vi "仁莫密封检测系统.vi"() -> ()   [LabVIEW 2020]
uses:
  <vilib>/NI/Modbus Library/API/Master/Modbus Master.lvclass
  <vilib>/Utility/file.llb/Read Delimited Spreadsheet (string).vi
  <vilib>/NI/Modbus Library/Transmission Data Unit/RTU/RTU Data Unit.lvclass
  <vilib>/NI/Modbus Library/Master Function Definition/Master Function Definition.lvclass
  <vilib>/NI/Modbus Library/Network Protocol/Network Master/Serial/Serial Master.lvclass
  <vilib>/event_ctls.llb/eventvkey.ctl
panel:
  in  "产品序号":string
  out "MES状态":bool
  out "通讯状态":bool
  out "刷新按钮":bool
  out "参数组别":string
  out "测试时间":string
  out "实时压力":string
  out "泄露压力":string
  out "门限压力":string
  out "目标压力":string
  out "测试 NG":string
  out "测试 OK":string
  out "测试结果":string
  out "测试总量":string
  out "实时压力(图)":dbl(graph)
  in  "清除计数":bool
  in  "设备启动":bool
  out "消息框":string
  in  "设备停止":bool
  in  "阻断通讯":bool=TRUE
  out "运行状态":string
  out "失败原因":string
  in  "Exit":bool
  # "仁 莫 密 封 检 测 系 统"
  # "S"
  # "Pa"
  # "Pa"
  # "Pa"
  # "Pa"
  # "pcs"
  # "pcs"
  # "pcs"
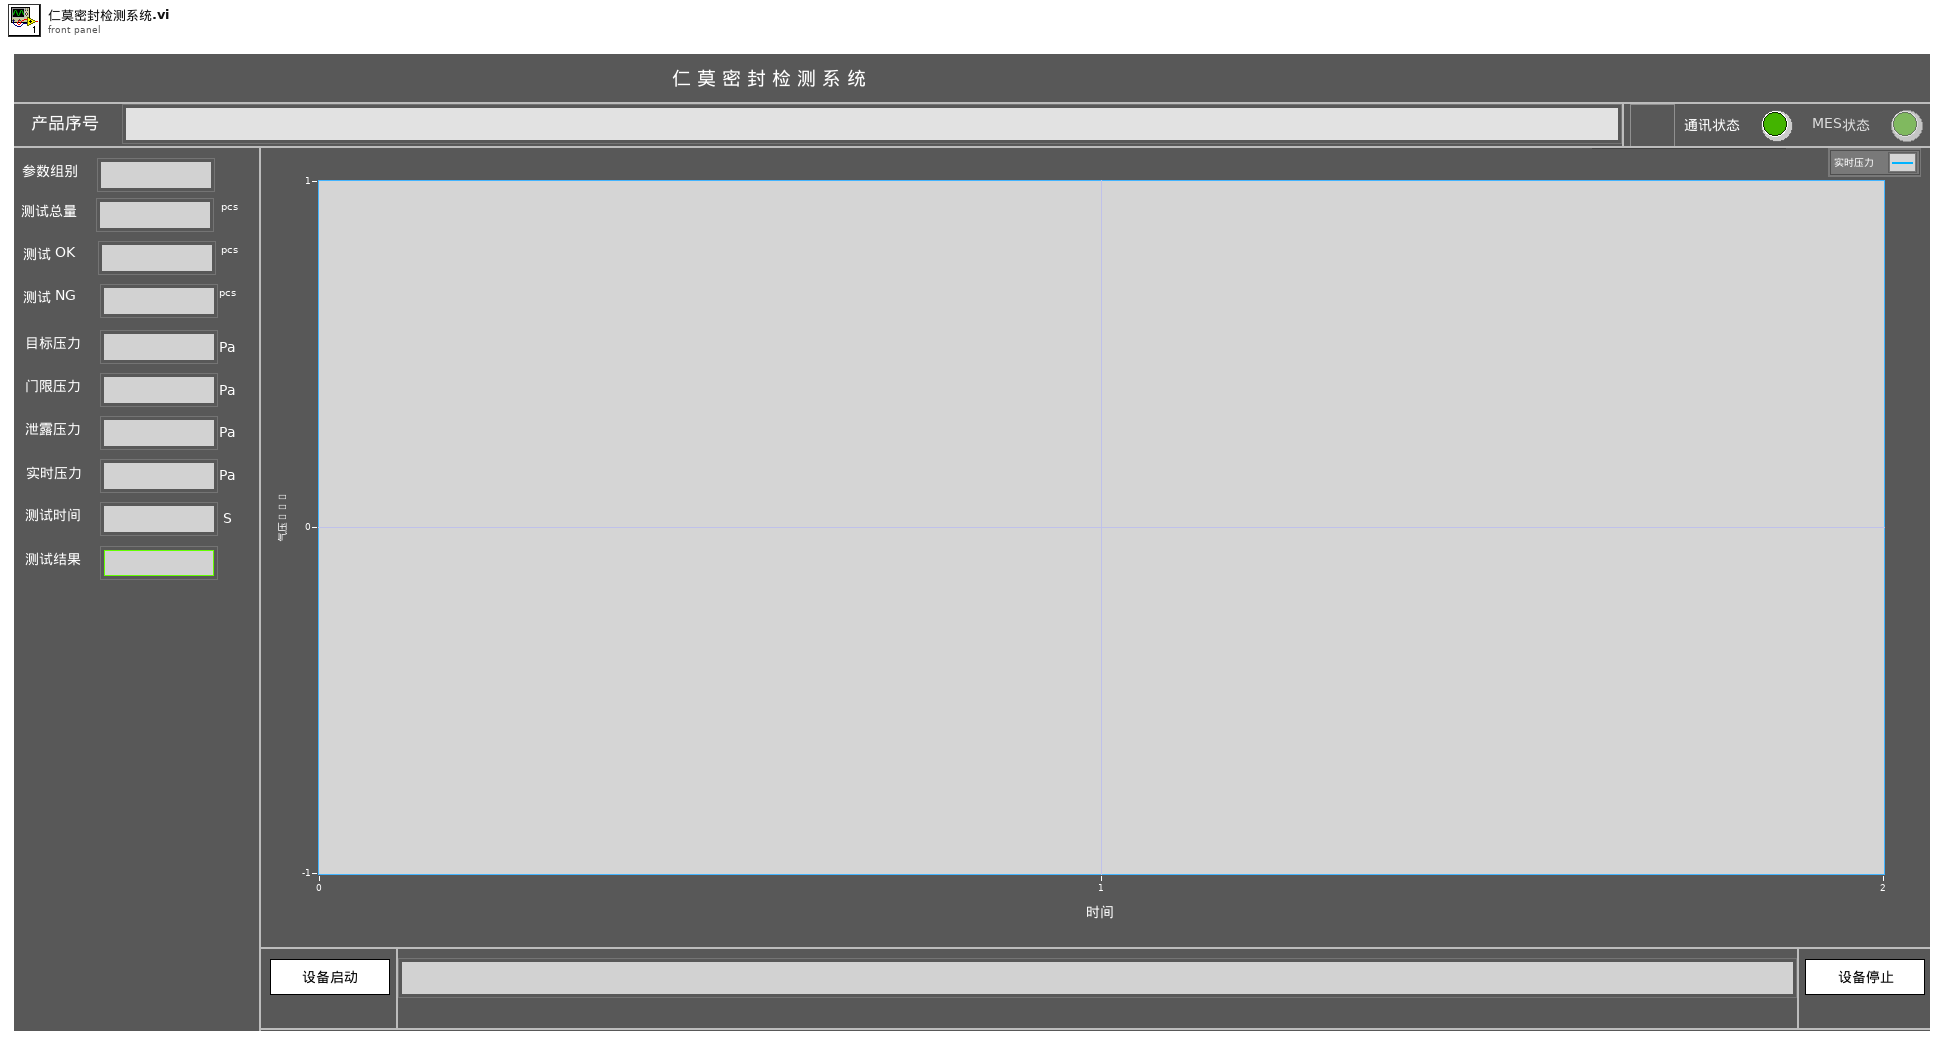
[diagram p1: front panel]
types:
  T1 = typedef "eventvkey.ctl" = enum16{"ASCII", "Enter", "Return", "Shift", "Ctrl", "Alt", "Cmd", "Opt", "Caps", "NumLock", "Clear", "Break", "Up", "Down", "Left", "Right", "Insert", "Delete", "Home", "End", "PageUp", "PageDown", "Escape", "Help", "Pause", "ScrollLock", "F1", "F2", "F3", "F4", "F5", "F6", "F7", "F8", "F9", "F10", "F11", "F12", "F13", "F14", "F15", "F16", "F17", "F18", "F19", "F20", "F21", "F22", "F23", "F24", "Play", "VolumeUp", "VolumeDown", "Mute", "Two Byte Char"}
  T2 = cluster{"地址":u16, "数量":u16, "寄存器值":u16[], "产品总数":string}[]
  T3 = enum32{"Invalid", "Standard", "Closed", "Hidden", "Minimized", "Maximized"}
  T4 = enum32{"invalid app kind", "Development System", "Run Time System", "Student Edition", "Embedded LabVIEW", "Evaluation", "Custom"}
  T5 = cluster{"地址":u16, "数量":u16, "寄存器值":u16[], "名称":string}[]
  T6 = cluster{"读取信息簇":cluster{"地址":u16, "数量":u16, "寄存器值":u16[], "名称":string}, "值解析":string}[]
  T7 = cluster{"温度instance":refnum<class "Modbus Master.lvclass">, "Core":cluster{"Current VI Reference":refnum<vi>, "Close Panel on Exit?":bool}, "serial master instance":refnum<class "Modbus Master.lvclass">, "进站OK":bool, "连接成功":bool, "正在运行":bool, "用户登录":bool, "A读保持寄存器信息组":cluster{"地址":u16, "数量":u16, "寄存器值":u16[], "名称":string}[], "A写入线圈信息组":cluster{"地址":u16, "布尔":bool, "名称":string}[], "A读多组线圈信息组":cluster{"地址":u16, "数量":u16, "名称":string, "线圈组":bool[]}[]}
  T8 = cluster{"连接成功":bool, "MB_实体":refnum<class "Modbus Master.lvclass">}
  T9 = cluster{"地址":u16, "数量":u16, "名称":string, "线圈组":bool[]}[]
  T10 = cluster{"Current VI Reference":refnum<vi>, "Close Panel on Exit?":bool}
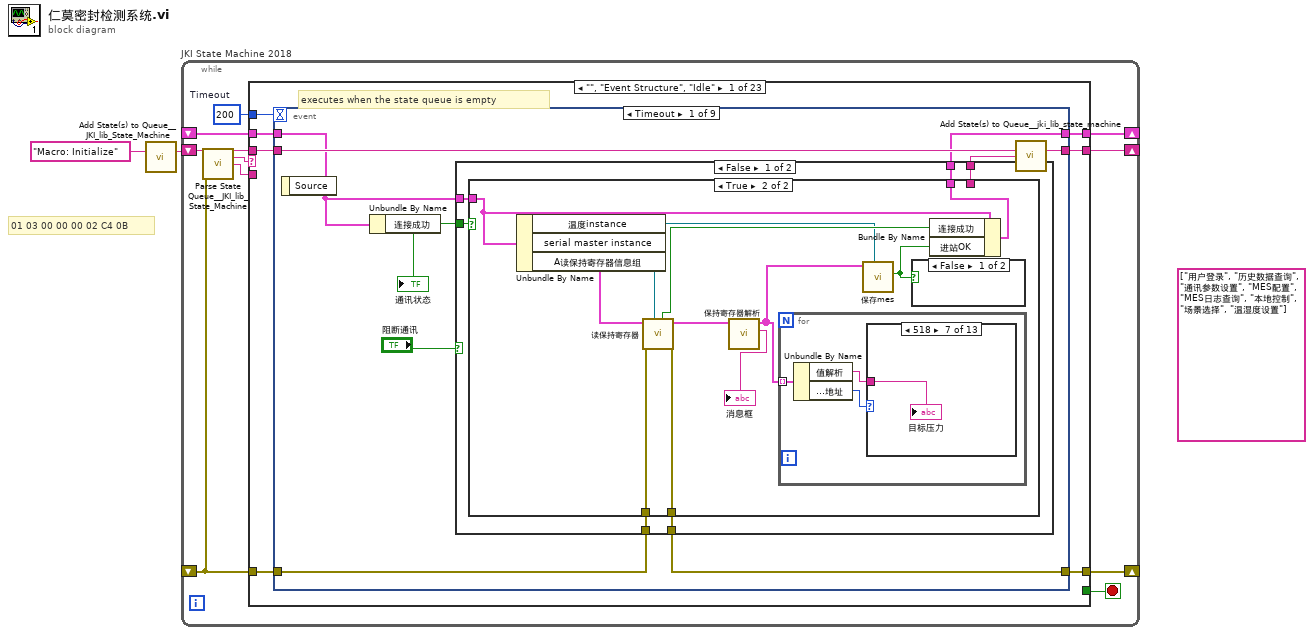
[diagram p0: block diagram]
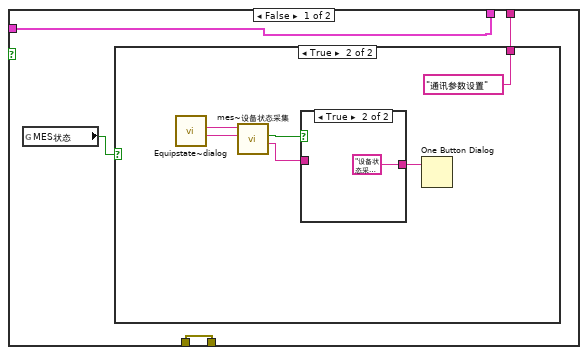
[diagram p2: hidden frame]
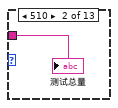
[diagram p7: hidden frame]
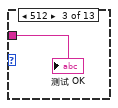
[diagram p8: hidden frame]
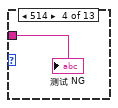
[diagram p9: hidden frame]
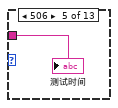
[diagram p10: hidden frame]
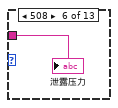
[diagram p11: hidden frame]
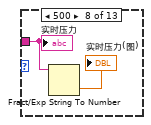
[diagram p12: hidden frame]
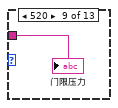
[diagram p13: hidden frame]
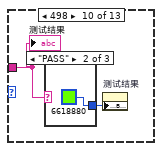
[diagram p14: hidden frame]
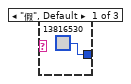
[diagram p15: hidden frame]
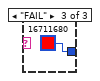
[diagram p16: hidden frame]
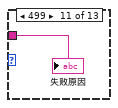
[diagram p17: hidden frame]
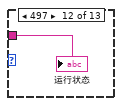
[diagram p18: hidden frame]
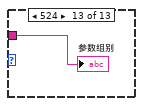
[diagram p19: hidden frame]
diagram:
  (unwired) string[] ["用户登录", "历史数据查询", "通讯参数设置", "MES配置", "MES日志查询", "本地控制", "场景选择", "温湿度设置"] ("L10n_item tags 1")
  # "01 03 00 00 00 02 C4 0B"
  n1 = call <vilib>:"Add State(s) to Queue__JKI_lib_State_Machine.vi"("State(s) in (\"\")"="Macro: Initialize") -> ("States Out"=w2:string)  [unwired: 14 in]
  n2 = while "JKI State Machine 2018" {
    shift-right: [w6] -> _
    shift-left: _ -> [w5]
    shift-right: [w9] -> _
    shift-left: _ -> [w3]
    shift-right: [w8] -> _
    shift-left: w2 -> [w10]
    stop <- w7 stop-if-true
    w4 = 200  # Timeout
    n3 = call <vilib>:"Parse State Queue__JKI_lib_State_Machine.vi"("State Queue"=w10, "Error In (no error)"=w3) -> ("Remaining States"=w12:string, "Current State"=w13:string, "Arguments"=w11:string)  [unwired: 11 in]
    n4 = case shown="\"\", \"Event Structure\", \"Idle\"" w13 {
      selector: w13 -> [_ _ w224 _ _ _ _ _ _ _ _ _ _ _ _ _ _ _ _ _ _ _ _]
      tunnel: w12 -> [w20 w223 w228 w247 w254 w259 w263 w284 w292 w296 w310 w316 w327 w396 w401 w411 w416 w432 w457 w506 w549 w561 w566]
      tunnel: w11 -> [_ _ _ _ _ _ _ _ _ _ _ w311 w321 _ _ _ _ _ _ _ _ _ _]
      tunnel: w5 -> [w18 w220 w226 w240 w251 w257 w260 _ w288 w293 w308 w314 w323 w393 w398 w408 w413 w426 w451 w500 w542 w558 w563]
      tunnel: [w17 w221 w230 w244 errorcluster {"status"=FALSE, "code"=0, "source"=""} ("error out") w256 w261 w281 w289 w294 w307 w312 w324 w394 w399 w409 w414 w422 w454 w503 w546 w559 w564] -> w9
      tunnel: w3 -> [w16 w221 w229 w244 w249 w256 w261 w281 w286 w294 w307 w313 w325 w394 w399 w409 w414 w429 w455 w504 w547 w559 w564]
      tunnel: [w19 w222 w227 w246 w253 w258 w262 w283 w291 w295 w309 w315 w326 w395 w400 w410 w415 w431 w456 w505 w548 w560 w565] -> w8
      tunnel: [_ _ _ _ _ TRUE _ _ _ _ _ _ _ _ _ _ _ _ _ _ _ _ _] -> w7
      tunnel: [w15 w220 w226 w245 w251 w257 w260 w282 w288 w293 w308 w314 w323 w393 w398 w408 w413 w424 w449 w498 w543 w558 w562] -> w6
      tunnel: w4 -> [w14 _ _ _ _ _ _ _ _ _ _ _ _ _ _ _ _ _ _ _ _ _ _]
      frame "", "Event Structure", "Idle" {
        # "executes when the state queue is empty"
        n5 = event shown="[0] Timeout" {
          selector: _ -> [_ _ _ _ _ _ _ _ _]
          dyn-events: _ -> [_ _ _ _ _ _ _ _ _]
          timeout: w14 -> [_ _ _ _ _ _ _ _ _]
          tunnel: w20 -> [w29 w86 w91 w97 w171 w193 w203 w213 w219]
          tunnel: [w28 w85 w90 w96 w170 w193 w202 w212 w218] -> w19
          tunnel: w18 -> [w27 w83 w88 w93 w168 w194 w198 w210 w216]
          tunnel: [w25 w84 w89 w95 w169 w191 w195 w211 w217] -> w17
          tunnel: w16 -> [w26 w84 w89 w95 w169 w191 w196 w211 w217]
          tunnel: [w24 w83 w88 w92 w167 w194 w197 w210 w216] -> w15
          event Timeout {
            n6 = event-data() -> ()  [unwired: 1 in, 1 out]
            n7 = Unbundle By Name(w27) -> ("连接成功"=w22:bool)
            "通讯状态" <- w22
            n8 = case shown="False" "阻断通讯" {
              tunnel: w22 -> [w35 _]
              tunnel: w27 -> [w34 w80]
              tunnel: w26 -> [w33 w81]
              tunnel: [w32 w81] -> w25
              tunnel: [w31 w80] -> w24
              tunnel: [w30 _] -> w21
              frame False {
                n9 = case shown="True" w35 {
                  tunnel: w34 -> [w37 w57]
                  tunnel: w33 -> [w39 w59]
                  tunnel: [w39 w58] -> w32
                  tunnel: [w37 w51] -> w31
                  tunnel: [w36 _] -> w30
                  frame False {
                    n10 = global read "Global.vi" "MES状态"() -> (w38:bool)
                    n11 = case shown="True" w38 {
                      tunnel: [_ "通讯参数设置"] -> w36
                      frame False {
                      }
                      frame True {
                        n12 = call "Equipstate~dialog.vi"() -> ("RecordDate"=w44:string, "Equipstate"=w45:string)  [unwired: 10 in]
                        n13 = call "mes~设备状态采集.vi"("RecordDate"=w44, "设备状态"=w45) -> ("ErrorMessage"=w42:string, "设备状态采集成功"=w43:bool)  [unwired: 7 in, 1 out]
                        n14 = case shown="True" w43 {
                          tunnel: w42 -> [w46 _]
                          tunnel: [w46 "设备状态采集成功。"] -> w41
                          frame False {
                          }
                          frame True {
                          }
                        }
                        n15 = One Button Dialog(message=w41) -> ()  [unwired: 1 in, 1 out]
                      }
                    }
                  }
                  frame True {
                    n16 = Unbundle By Name(w57) -> ("温度instance"=w48:refnum<class "Modbus Master.lvclass">, "serial master instance"=w56:refnum<class "Modbus Master.lvclass">, "A读保持寄存器信息组"=w55:T5)
                    n17 = call "读保持寄存器.vi"("MB_实体"=w56, "error in"=w59, "读保持寄存器信息组__输入"=w55) -> ("输出簇"=w58:errorcluster, "读保持寄存器信息组_输出"=w53:T5, "连接成功"=w54:bool)  [unwired: 6 in]
                    n18 = call "保持寄存器解析.vi"("A读保持寄存器信息组"=w53) -> ("运行状态"=→"消息框":string, "参数值"=w50:T6)  [unwired: 9 in]
                    n19 = for {
                      tunnel: w50 -> [w61] mode=indexing
                      n20 = Unbundle By Name(w61) -> ("值解析"=w60:string, "读取信息簇.地址"=w62:u16)
                      n21 = case shown="518" w62 {
                        tunnel: w60 -> [_ w63 w64 w65 w66 w67 w68 w70 w71 w73 w77 w78 w79]
                        frame Default {
                        }
                        frame 510 {
                          "测试总量" <- w63
                        }
                        frame 512 {
                          "测试 OK" <- w64
                        }
                        frame 514 {
                          "测试 NG" <- w65
                        }
                        frame 506 {
                          "测试时间" <- w66
                        }
                        frame 508 {
                          "泄露压力" <- w67
                        }
                        frame 518 {
                          "目标压力" <- w68
                        }
                        frame 500 {
                          n22 = Fract/Exp String To Number(string=w70) -> (number=→"实时压力(图)":dbl)  [unwired: 3 in, 1 out]
                          "实时压力" <- w70
                        }
                        frame 520 {
                          "门限压力" <- w71
                        }
                        frame 498 {
                          n23 = case shown="\"PASS\"" w73 {
                            tunnel: [u32 13816530 ("颜色盒") u32 6618880 u32 16711680] -> w72
                            frame "假", Default {
                            }
                            frame "PASS" {
                            }
                            frame "FAIL" {
                            }
                          }
                          n24 = property on="测试结果" class="Str"("Text.BGColor"=w72) -> ()  [unwired: 2 in, 2 out]
                          "测试结果" <- w73
                        }
                        frame 499 {
                          "失败原因" <- w77
                        }
                        frame 497 {
                          "运行状态" <- w78
                        }
                        frame 524 {
                          "参数组别" <- w79
                        }
                      }
                    }
                    n25 = call "保存mes.vi"("温度instance"=w48, "参数值"=w50) -> ("进站OK?"=w49:bool)  [unwired: 9 in]
                    n26 = case shown="False" w49 {
                      frame False {
                      }
                      frame True {
                      }
                    }
                    n27 = Bundle By Name(cluster=w57, "连接成功"=w54, "进站OK"=w49) -> (w51:T7)
                  }
                }
              }
              frame True {
              }
            }
            n28 = call <vilib>:"Add State(s) to Queue__jki_lib_state_machine.vi"("State(s) in (\"\")"=w29, "State(s) at Back (\"\")"=w21) -> ("States Out"=w28:string)  [unwired: 13 in]
          }
          event "设备启动": Value Change {
            n29 = event-data() -> ()  [unwired: 1 in, 1 out]
            n30 = call <vilib>:"Add State(s) to Queue__jki_lib_state_machine.vi"("State(s) in Front (\"\")"="//Communication: 读运行标志\nCommunication: 设备启动\n//Communication: 读运行标志", "State(s) in (\"\")"=w86) -> ("States Out"=w85:string)  [unwired: 13 in]
          }
          event "设备停止": Value Change {
            n31 = event-data() -> ()  [unwired: 1 in, 1 out]
            n32 = call <vilib>:"Add State(s) to Queue__jki_lib_state_machine.vi"("State(s) in Front (\"\")"="//Communication: 读运行标志\nCommunication: 设备停止\n//Communication: 读运行标志", "State(s) in (\"\")"=w91) -> ("States Out"=w90:string)  [unwired: 13 in]
          }
          event Menu Selection (User) {
            n33 = event-data() -> ("ItemTag"=w94:string)  [unwired: 1 in]
            n34 = case shown="\"本地控制\"" w94 {
              tunnel: w93 -> [w98 w101 w109 w120 w132 w134 w145 w158 w163]
              tunnel: [w98 w100 w109 w120 w132 w133 w144 w158 w162] -> w92
              frame "假", Default {
              }
              frame "用户登录" {
                n35 = call "mes~Login Dialog.vi"() -> ("Success?"=w99:bool)  [unwired: 10 in, 1 out]
                n36 = Bundle By Name(cluster=w101, "用户登录"=w99) -> (w100:T7)
                n37 = case shown="True" w99 {
                  frame False {
                    n38 = Current VI's Menubar() -> (w103:refnum<k9>)
                    n39 = Delete Menu Items(9:w103) -> (3:w102:refnum<k9>)  [unwired: 3 in, 1 out]
                    n40 = Insert Menu Items(7:string[] ["用户登录", "历史数据查询", "MES配置", "MES日志查询", "本地控制", "温湿度设置"] ("L10n_item tags 1"), 9:w102) -> ()  [unwired: 4 in, 3 out]
                  }
                  frame True {
                    n41 = Current VI's Menubar() -> (w107:refnum<k9>)
                    n42 = Delete Menu Items(9:w107) -> (0:w105:errorcluster, 3:w106:refnum<k9>)  [unwired: 3 in]
                    n43 = Insert Menu Items(6:w105, 7:string[] ["用户登录", "历史数据查询", "通讯参数设置", "MES配置", "MES日志查询", "本地控制"] ("L10n_item tags 1"), 9:w106) -> ()  [unwired: 3 in, 3 out]
                  }
                }
              }
              frame "历史数据查询" {
                n44 = stacked-sequence {
                  frame #0 {
                    n45 = call <vilib>:"Check if File or Folder Exists.vi"("path"=path "D:/MES" ("路径")) -> ("file or folder exists?"=w112:bool, "dup path"=w111:path)  [unwired: 8 in, 1 out]
                    n46 = case shown="False" w112 {
                      tunnel: w111 -> [w114 w115]
                      tunnel: [w113 w115] -> _
                      frame False {
                        n47 = Create Folder(path (use dialog)=w114) -> (created path=w113:path)  [unwired: 2 in, 2 out]
                      }
                      frame True {
                      }
                    }
                  }
                  frame #1 {
                    n48 = call <vilib>:"Space Constant.vi"() -> ("String"=w117:string)
                    n49 = Concatenate Strings("explorer" ("字符串"), w117, "D:\\MES" ("字符串")) -> (w119:string)
                    n50 = call <vilib>:"System Exec.vi"("command line"=w119) -> ()  [unwired: 7 in, 4 out]
                  }
                }
              }
              frame "MES日志查询" {
                n51 = stacked-sequence {
                  frame #0 {
                    n52 = call <vilib>:"Check if File or Folder Exists.vi"("path"=path "D:/Log" ("路径")) -> ("file or folder exists?"=w123:bool, "dup path"=w122:path)  [unwired: 8 in, 1 out]
                    n53 = case shown="False" w123 {
                      tunnel: w122 -> [w125 w126]
                      tunnel: [w124 w126] -> _
                      frame False {
                        n54 = Create Folder(path (use dialog)=w125) -> (created path=w124:path)  [unwired: 2 in, 2 out]
                      }
                      frame True {
                      }
                    }
                  }
                  frame #1 {
                    n55 = call <vilib>:"Space Constant.vi"() -> ("String"=w128:string)
                    n56 = Concatenate Strings("explorer" ("字符串"), w128, "D:\\Log" ("字符串")) -> (w130:string)
                    n57 = call <vilib>:"System Exec.vi"("command line"=w130) -> ()  [unwired: 7 in, 4 out]
                  }
                }
              }
              frame "MES配置" {
                n58 = call "mes配置前验证.vi"() -> ("Success?"=w131:bool)  [unwired: 10 in, 1 out]
                n59 = case shown="True" w131 {
                  frame False {
                  }
                  frame True {
                    n60 = call "mes参数配置.vi"() -> ()  [unwired: 11 in, 1 out]
                  }
                }
              }
              frame "通讯参数设置" {
                n61 = stacked-sequence {
                  tunnel: w134 -> [_ w139 _]
                  tunnel: [_ w136 _] -> w133
                  frame #0 {
                    n62 = local write "阻断通讯"(TRUE ("阻断通讯")) -> ()
                  }
                  frame #1 {
                    n63 = call "通讯参数设置.vi"() -> ("A设备簇"=w140:T8)  [unwired: 5 in]
                    n64 = Unbundle By Name(w140) -> ("MB_实体"=w138:refnum<class "Modbus Master.lvclass">, "连接成功"=w137:bool)
                    n65 = Bundle By Name(cluster=w139, "serial master instance"=w138, "连接成功"=w137) -> (w136:T7)
                  }
                  frame #2 {
                    n66 = local write "阻断通讯"(FALSE ("阻断通讯")) -> ()
                  }
                }
              }
              frame "本地控制" {
                n67 = call "本地控制.vi"() -> ("远程2"=w143:bool)  [unwired: 11 in]
                "MES状态" <- w143
                n68 = Not(x=w143) -> (.not. x?=w142:bool)
                n69 = Bundle By Name(cluster=w145, "用户登录"=w142, "进站OK"=w142) -> (w144:T7)
                n70 = global write "Global.vi" "MES状态"(w143) -> ()
                n71 = global write "Global.vi" "产品进站"(w142) -> ()
                n72 = case shown="True" w143 {
                  frame False {
                    n73 = Current VI's Menubar() -> (w147:refnum<k9>)
                    n74 = Delete Menu Items(9:w147) -> (3:w146:refnum<k9>)  [unwired: 3 in, 1 out]
                    n75 = Insert Menu Items(7:string[] ["历史数据查询", "通讯参数设置", "MES配置", "MES日志查询", "本地控制"] ("L10n_item tags 1"), 9:w146) -> ()  [unwired: 4 in, 3 out]
                  }
                  frame True {
                    n76 = Current VI's Menubar() -> (w151:refnum<k9>)
                    n77 = Delete Menu Items(9:w151) -> (0:w149:errorcluster, 3:w150:refnum<k9>)  [unwired: 3 in]
                    n78 = Insert Menu Items(6:w149, 7:string[] ["用户登录", "历史数据查询", "通讯参数设置", "MES配置", "MES日志查询", "本地控制"] ("L10n_item tags 1"), 9:w150) -> ()  [unwired: 3 in, 3 out]
                  }
                }
              }
              frame "场景选择" {
                n79 = call "Equipstate~dialog.vi"() -> ("RecordDate"=w156:string, "Equipstate"=w157:string)  [unwired: 10 in]
                n80 = call "mes~设备状态采集.vi"("RecordDate"=w156, "设备状态"=w157) -> ("ErrorMessage"=w154:string, "设备状态采集成功"=w155:bool)  [unwired: 7 in, 1 out]
                n81 = case shown="True" w155 {
                  tunnel: w154 -> [w159 _]
                  tunnel: [w159 "设备状态采集正常。"] -> w153
                  frame False {
                  }
                  frame True {
                  }
                }
                n82 = One Button Dialog(message=w153) -> ()  [unwired: 1 in, 1 out]
              }
              frame "温湿度设置" {
                n83 = call "通讯参数设置.vi"("波特率"=u32 9600) -> ("A设备簇"=w165:T8)  [unwired: 4 in]
                n84 = Unbundle By Name(w165) -> ("MB_实体"=w164:refnum<class "Modbus Master.lvclass">)
                n85 = Bundle By Name(cluster=w163, "温度instance"=w164) -> (w162:T7)
              }
            }
            n86 = call <vilib>:"Add State(s) to Queue__jki_lib_state_machine.vi"("State(s) in (\"\")"=w97) -> ("States Out"=w96:string)  [unwired: 14 in]
          }
          event "产品序号": Key Down {
            n87 = event-data() -> ("VKey"=w166:T1)  [unwired: 1 in]
            n88 = disable-structure shown="Disabled" {
              disable-tunnel: w168 -> [w177 w190]
              disable-tunnel: [w176 w190] -> w167
              disable-tunnel: w166 -> [w174 _]
              frame Disabled {
                n89 = Equal?(x=w174, y=eventvkey."Return" ("V键")) -> (x = y?=w172:bool)
                n90 = case shown="False" w172 {
                  tunnel: [FALSE ("进站成功") w180] -> w175
                  frame False {
                  }
                  frame True {
                    n91 = global read "Global.vi" "MES状态"() -> (w181:bool)
                    n92 = case shown="True" w181 {
                      tunnel: "产品序号" -> [_ w187]
                      tunnel: [TRUE ("进站成功") w186] -> w180
                      frame False {
                      }
                      frame True {
                        n93 = call "mes~产品进站.vi"("identification"=w187) -> ("ErrorMessage"=w185:string, "进站成功"=w186:bool)  [unwired: 8 in, 1 out]
                        n94 = case shown="False" w186 {
                          tunnel: w185 -> [_ _]
                          tunnel: ["产品进站失败。" "产品进站成功。"] -> w184
                          frame False {
                          }
                          frame True {
                          }
                        }
                        n95 = One Button Dialog(message=w184) -> ()  [unwired: 1 in, 1 out]
                      }
                    }
                    n96 = global write "Global.vi" "PACK编码"("产品序号") -> ()
                  }
                }
                n97 = global write "Global.vi" "产品进站"(w175) -> ()
                n98 = Bundle By Name(cluster=w177, "进站OK"=w175) -> (w176:T7)
                "刷新按钮" <- FALSE ("刷新按钮")
              }
              frame Enabled {
              }
            }
            n99 = call <vilib>:"Add State(s) to Queue__jki_lib_state_machine.vi"("State(s) in (\"\")"=w171) -> ("States Out"=w170:string)  [unwired: 14 in]
          }
          event "产品序号": Value Change {
            n100 = event-data() -> ()  [unwired: 1 in, 1 out]
            n101 = local read "产品序号"() -> (w192:string)
            n102 = global write "Global.vi" "PACK编码"(w192) -> ()
          }
          event "清除计数": Value Change {
            n103 = event-data() -> ()  [unwired: 1 in, 1 out]
            n104 = local write "清除计数"(FALSE) -> ()
            n105 = Unbundle By Name(w198) -> ("serial master instance"=w199:refnum<class "Modbus Master.lvclass">)
            n106 = disable-structure shown="Disabled" {
              disable-tunnel: [w208 _] -> w200
              disable-tunnel: w199 -> [w207 _]
              disable-tunnel: w196 -> [w205 _]
              disable-tunnel: [w204 _] -> w195
              frame Disabled {
                n107 = call "写保持寄存器.vi"("MB_实体"=w207, "error in"=w205, "读保持寄存器信息组__输入"=T2 [{"地址"=510, "数量"=2, "寄存器值"=[0, 0], "产品总数"="产品总数"}, {"地址"=512, "数量"=2, "寄存器值"=[0, 0], "产品总数"="合格数量"}, {"地址"=514, "数量"=2, "寄存器值"=[0, 0], "产品总数"="泄露数量"}]) -> ("输出簇"=w204:errorcluster, "连接成功"=w208:bool)  [unwired: 7 in]
              }
              frame Enabled {
              }
            }
            n108 = Bundle By Name(cluster=w198, "连接成功"=w200) -> (w197:T7)
            n109 = call <vilib>:"Add State(s) to Queue__jki_lib_state_machine.vi"("State(s) in (\"\")"=w203) -> ("States Out"=w202:string)  [unwired: 14 in]
          }
          event "Exit": Value Change {
            # "Exit Button Value Change (pressed) Event\n(this executes Macro: Exit to terminate the VI)"
            n110 = event-data() -> ()  [unwired: 1 in, 1 out]
            n111 = call <vilib>:"Add State(s) to Queue__jki_lib_state_machine.vi"("State(s) in Front (\"\")"="Macro: Exit", "State(s) in (\"\")"=w213) -> ("States Out"=w212:string)  [unwired: 13 in]
          }
          event Panel Close? {
            # "Discard the event because we'll close the front panel ourselves in Macro: Exit"
            # "Close Panel button (pressed) Event\n(this executes Macro: Exit to terminate the VI)"
            n112 = event-data() -> ()  [unwired: 1 in, 1 out]
            n113 = event-data("Discard?"=TRUE) -> ()  [unwired: 1 in, 1 out]
            n114 = call <vilib>:"Add State(s) to Queue__jki_lib_state_machine.vi"("State(s) in Front (\"\")"="Macro: Exit", "State(s) in (\"\")"=w219) -> ("States Out"=w218:string)  [unwired: 13 in]
          }
        }
      }
      frame "---------- Core ----------" {
        # "Do not put any code in this frame.\n(it is a separator no-op)"
        n115 = call <vilib>:"Add State(s) to Queue__jki_lib_state_machine.vi"("State(s) in (\"\")"=w223) -> ("States Out"=w222:string)  [unwired: 14 in]
      }
      frame Default {
        w233 = 42 items=["No error", "Argument error", "Memory is full", "Out of zone", "End of file", "File already open", "Generic file I/O error", "File not found", "File permission error", "Disk is full", "Duplicate path", "Too many files open", "System feature not enabled", "Resource file not found", "Cannot add resource", "Resource not found", "Image not found", "Image memory error", "Pen does not exist", "Config type invalid", "Config token not found", "Config parse error", "Config memory error", "Bad external code format", "Bad external code offset", "External code not present", "Null window", "Destroy window error", "Null menu", "Print aborted", "Bad print record", "Print driver error", "Windows error during printing", "Memory error during printing", "Print dialog error", "Generic print error", "Invalid device refnum", "Device not found", "Device parameter error", "Device unit error", "Cannot open device", "Device call aborted", "Generic error", "Cancelled by user", "Object ID too low", "Object ID too high", "Object not in heap", "Unknown heap", "Unknown object (invalid DefProc)", "Unknown object (DefProc not in table)", "Message out of range", "Invalid (null) method", "Unknown message", "Manager call not supported", "Bad address", "Network operation in progress", "Network operation timed out", "Connection is busy", "Network attribute not supported", "Network error", "Address in use", "System out of memory", "Connection aborted", "Connection refused", "Not connected", "Already connected", "Connection closed", "Initialization error (interapplication manager)", "Bad occurrence", "Wait on unbound occurrence handler", "Occurrence queue overflow", "Datalog type conflict", "Unused", "Unrecognized type (interapplication manager)", "Memory corrupt", "Failed to make temporary DLL", "Old CIN version", "Drag socket not found", "Failed to load drop-object", "Failed to register OLE object", "Failed to release OLE object", "Format specifier type mismatch", "Unknown format specifier", "Too few format specifiers", "Too many format specifiers", "Scan failed", "Newer CIN version", "Error converting to variant", "Runtime menu error", "Password tampered", "Variant attribute not found", "Incompatible variant data type", "Event data is not available", "Event Store is not present", "Occurrence is not found", "Event Queue is not created", "Event info is not available", "Refnum passed is NULL", "Error retrieving Class GUID", "Error retrieving CoClass GUID", "Error retrieving TypeLib GUID.", "Bad built application magic bytes.", "Specific driver is different from the specific driver associated with the Logical Name.", "There is no session opened to the class driver.", "Max Error", "MAX - Error with config objects", "MAX - Error loading configuration", "MAX - Group not supported"]
        # "Current State"
        # "Do not delete, rename, or modify this frame.\n(this is used to capture unhandled states and typos)"
        # "Handle mistyped state name (developer tool)"
        n116 = Format Into String(format string="Software Exception: Unhandled State \"%s\"." ("message"), error in=w229, w224) -> (resulting string=w232:string, error out=w231:errorcluster)  [unwired: 1 in]
        n117 = call <vilib>:"Error Cluster From Error Code.vi"("show call chain? (False)"=TRUE, "error in (no error)"=w231, "error message (\"\")"=w232, "error code (0)"=w233) -> ("error out"=w230:errorcluster)  [unwired: 5 in]
        n118 = call <vilib>:"Add State(s) to Queue__jki_lib_state_machine.vi"("State(s) in (\"\")"=w228) -> ("States Out"=w227:string)  [unwired: 14 in]
      }
      frame "Initialize Core Data" {
        # "Do not delete, rename, or modify this frame.\n(this is used to determine panel behavior on exit)"
        # "originally closed?"
        # "exe?"
        # "If panel starts closed or is an EXE, then close it when we exit"
        n119 = property class="VI"() -> ("FP.State"=w237:T3)  [unwired: 2 in, 2 out]
        n120 = property class="App"() -> ("App.Kind"=w243:T4)  [unwired: 2 in, 2 out]
        n121 = control-ref of="Current VI Reference"() -> (w238:refnum<vi>)
        n122 = Equal?(x=w237, y=T3."Closed" ("Front Panel Window:State")) -> (x = y?=w235:bool)
        n123 = Equal?(x=w243, y=T4."Run Time System" ("Application:Kind")) -> (x = y?=w241:bool)
        n124 = Or(x=w235, y=w241) -> (x .or. y?=w239:bool)
        n125 = Bundle By Name(cluster=w240, "Core.Current VI Reference"=w238, "Core.Close Panel on Exit?"=w239) -> (w245:T7)
        n126 = call <vilib>:"Add State(s) to Queue__jki_lib_state_machine.vi"("State(s) in (\"\")"=w247) -> ("States Out"=w246:string)  [unwired: 14 in]
      }
      frame "Error Handler" {
        # "Handle any errors here.\nYou can also output any states to clean-up after errors occur"
        # "Clear error"
        n127 = Unbundle By Name(w249) -> ("source"=w248:string)
        n128 = One Button Dialog(message=w248) -> ()  [unwired: 1 in, 1 out]
        n129 = call <vilib>:"Add State(s) to Queue__jki_lib_state_machine.vi"("State(s) in Front (\"\")"="/* Post Error States", "State(s) in (\"\")"=w254) -> ("States Out"=w253:string)  [unwired: 13 in]
      }
      frame "Exit" {
        # "Do not put any code in this frame.\n(No errors that occur here will be handled.)"
        n130 = call <vilib>:"Add State(s) to Queue__jki_lib_state_machine.vi"("State(s) in (\"\")"=w259) -> ("States Out"=w258:string)  [unwired: 14 in]
      }
      frame "---------- Data ----------" {
        # "Do not put any code in this frame.\n(It is a separator no-op. You can make a copy of this frame to create a new Data frame)"
        n131 = call <vilib>:"Add State(s) to Queue__jki_lib_state_machine.vi"("State(s) in (\"\")"=w263) -> ("States Out"=w262:string)  [unwired: 14 in]
      }
      frame "Data: Initialize" {
        w264 = refnum<class "Modbus Master.lvclass"> refnum  # 温度instance
        w265 = FALSE ("MES状态")
        w266 = FALSE  # 进站OK
        w273 = TRUE  # 用户登录
        w274 = FALSE  # 正在运行
        w275 = T5 [{"地址"=510, "数量"=2, "寄存器值"=[0, 0], "名称"="产品总数"}, {"地址"=512, "数量"=2, "寄存器值"=[0, 0], "名称"="合格数量"}, {"地址"=514, "数量"=2, "寄存器值"=[0, 0], "名称"="泄露数量"}, {"地址"=506, "数量"=2, "寄存器值"=[0, 0], "名称"="1测试时间"}, {"地址"=508, "数量"=2, "寄存器值"=[0, 0], "名称"="1测试泄漏"}, {"地址"=518, "数量"=2, "寄存器值"=[0, 0], "名称"="1#目标压力"}, {"地址"=498, "数量"=1, "寄存器值"=[0, 0], "名称"="1#测试结果"}, {"地址"=500, "数量"=2, "寄存器值"=[0, 0], "名称"="实时压力"}, {"地址"=520, "数量"=2, "寄存器值"=[], "名称"="门限压力"}, {"地址"=499, "数量"=1, "寄存器值"=[], "名称"="失败原因"}, {"地址"=497, "数量"=1, "寄存器值"=[], "名称"="运行状态"}, {"地址"=524, "数量"=2, "寄存器值"=[], "名称"="参数组别"}]  # A读保持寄存器信息组
        w276 = T9 [{"地址"=507, "数量"=1, "名称"="1测试结束标志", "线圈组"=[FALSE, TRUE]}]  # A读多组线圈信息组
        w277 = cluster{"地址":u16, "布尔":bool, "名称":string}[] [{"地址"=50, "布尔"=FALSE, "名称"="启动"}, {"地址"=51, "布尔"=FALSE, "名称"="停止"}]  # A写入线圈信息组
        w278 = FALSE  # 连接成功
        w279 = refnum<class "Modbus Master.lvclass"> refnum  # serial master instance
        w280 = T10 {"Current VI Reference"=refnum, "Close Panel on Exit?"=FALSE}  # Core
        # "Initialize the shift-register data, here.\n(data names are defined by what you wire into the bundle function)"
        n132 = call <vilib>:"Application Directory.vi"() -> ("Application Directory"=w271:path)
        n133 = Build Path(base path=w271, name or relative path=path "data/mes.cfg") -> (appended path=w272:path)
        n134 = call-poly <vilib>:"Read Delimited Spreadsheet.vi"("file path (dialog if empty)"=w272, "delimiter (\\t)"="::" ("delimiter (\\t)")) -> ("all rows"=w267:string[][])  [unwired: 8 in, 5 out]
        n135 = call "mes初始化.vi"("mes"=w267) -> ()  [unwired: 11 in]
        n136 = global write "Global.vi" "MES状态"(w265) -> ()
        n137 = global write "Global.vi" "正在运行"(w265) -> ()
        n138 = local write "MES状态"(w265) -> ()
        n139 = global write "Global.vi" "产品进站"(w265) -> ()
        n140 = global write "Global.vi" "运行状态时间点"(dbl[] [0.0, 0.0, 0.0, 0.0, 0.0, 0.0, 0.0, 0.0, 0.0] ("运行状态时间点")) -> ()
        n141 = Bundle("温度instance"=w264, "Core"=w280, "serial master instance"=w279, "进站OK"=w266, "连接成功"=w278, "正在运行"=w274, "用户登录"=w273, "A读保持寄存器信息组"=w275, "A写入线圈信息组"=w277, "A读多组线圈信息组"=w276) -> (w282:T7)  [unwired: 1 in]
        n142 = call <vilib>:"Add State(s) to Queue__jki_lib_state_machine.vi"("State(s) in (\"\")"=w284) -> ("States Out"=w283:string)  [unwired: 14 in]
      }
      frame "Data: Cleanup" {
        # "Cleanup any data and references, here.\n(this is called automatically, by the Macro: Exit)"
        n143 = Unbundle By Name(w288) -> ("Core.Current VI Reference"=w290:refnum<vi>, "serial master instance"=w287:refnum<class "Modbus Master.lvclass">)
        n144 = call-dynamic "Shutdown.vi"("error in"=w286, "Modbus master in"=w287) -> ("error out"=w285:errorcluster)  [unwired: 9 in]
        n145 = Close Reference(reference=w290, error in (no error)=w285) -> (error out=w289:errorcluster)
        n146 = call <vilib>:"Add State(s) to Queue__jki_lib_state_machine.vi"("State(s) in (\"\")"=w292) -> ("States Out"=w291:string)  [unwired: 14 in]
      }
      frame "---------- UI ----------" {
        # "Do not put any code in this frame.\n(It is a separator no-op. You can make a copy of this frame to create a new UI frame)"
        n147 = call <vilib>:"Add State(s) to Queue__jki_lib_state_machine.vi"("State(s) in (\"\")"=w296) -> ("States Out"=w295:string)  [unwired: 14 in]
      }
      frame "UI: Initialize" {
        (unwired) "MES日志查询" ("L10n_menu item")
        (unwired) "MES配置" ("L10n_menu item")
        (unwired) "本地控制" ("L10n_menu item")
        w303 = ""
        # "Initialize the User Interface, here.\n(this is called automatically, by the Macro: Init)"
        n148 = call "读取配置文件.vi"("配置"="程序名") -> ("error out"=w302:errorcluster, "路径"=w301:string)  [unwired: 9 in]
        n149 = property class="VI"(error in=w302, "Front Panel.Title"=w301) -> (error out=w299:errorcluster)  [unwired: 1 in, 1 out]
        n150 = Current VI's Menubar() -> (w306:refnum<k9>)
        n151 = Delete Menu Items(6:w299, 9:w306) -> (0:w305:errorcluster, 3:w304:refnum<k9>)  [unwired: 2 in]
        n152 = local write "产品序号"(w303) -> ()
        n153 = global write "Global.vi" "PACK编码"(w303) -> ()
        n154 = Insert Menu Items(6:w305, 7:string[] ["历史数据查询", "通讯参数设置"] ("L10n_item tags 1"), 9:w304) -> ()  [unwired: 3 in, 3 out]
        n155 = property on="测试结果" class="Str"("Text.BGColor"=u32 13816530 ("颜色盒")) -> ()  [unwired: 2 in, 2 out]
        n156 = call <vilib>:"Add State(s) to Queue__jki_lib_state_machine.vi"("State(s) in (\"\")"=w310) -> ("States Out"=w309:string)  [unwired: 14 in]
      }
      frame "UI: Cursor Set" {
        # "Argument"
        # "Set and Unset Cursor Busy.\n(Usage: \"UI: Cursor Set >> Busy|Idle\")"
        n157 = case shown="\"Idle\", Default" w311 {
          tunnel: w313 -> [w318 w320]
          tunnel: [w317 w319] -> w312
          frame "Idle", Default {
            n158 = call <vilib>:"Unset Busy.vi"("error in (no error)"=w318) -> ("error out"=w317:errorcluster)  [unwired: 10 in]
          }
          frame "Busy" {
            n159 = call <vilib>:"Set Busy.vi"("error in (no error)"=w320) -> ("error out"=w319:errorcluster)  [unwired: 9 in, 1 out]
          }
        }
        n160 = call <vilib>:"Add State(s) to Queue__jki_lib_state_machine.vi"("State(s) in (\"\")"=w316) -> ("States Out"=w315:string)  [unwired: 14 in]
      }
      frame "UI: Front Panel State" {
        # "Argument"
        # "Set Front Panel Open or Closed\n(Usage: \"UI: Front Panel State >> Open|Close\")"
        n161 = Unbundle By Name(w323) -> ("Core.Current VI Reference"=w322:refnum<vi>)
        n162 = case shown="\"Maximize\", \"Maximized\"" w321 {
          tunnel: w325 -> [w333 w348 w359 w372 w385]
          tunnel: [w335 w349 w361 w374 w387] -> w324
          tunnel: w322 -> [w334 w346 w360 w373 w386]
          frame "Open", "Standard", Default {
            w328 = T3."Standard" ("State")
            n163 = property class="VI"(reference=w334, error in=w333) -> (reference out=w331:refnum<vi>, error out=w332:errorcluster, "FP.State"=w330:T3)
            n164 = Not Equal?(x=w330, y=w328) -> (x != y?=w329:bool)
            n165 = case shown="True" w329 {
              tunnel: [w339 w341] -> w335
              tunnel: w332 -> [w338 w341]
              tunnel: w331 -> [w337 _]
              tunnel: w328 -> [w336 _]
              frame True {
                n166 = invoke class="VI" method="FP.Open"(reference=w337, error in=w338, "Activate"=TRUE, "State"=w336) -> (error out=w339:errorcluster)  [unwired: 1 in, 4 out]
              }
              frame False {
              }
            }
          }
          frame "Close", "Closed" {
            n167 = property class="VI"(reference=w346, error in=w348) -> (reference out=w345:refnum<vi>, error out=w347:errorcluster, "FP.State"=w343:T3)
            n168 = Not Equal?(x=w343, y=T3."Closed" ("Front Panel Window:State")) -> (x != y?=w342:bool)
            n169 = case shown="True" w342 {
              tunnel: [w350 w353] -> w349
              tunnel: w347 -> [w350 w352]
              tunnel: w345 -> [_ w351]
              frame False {
              }
              frame True {
                n170 = invoke class="VI" method="FP.Close"(reference=w351, error in=w352) -> (error out=w353:errorcluster)  [unwired: 1 in, 2 out]
              }
            }
          }
          frame "Hidden", "Hide" {
            w354 = T3."Hidden" ("State")
            n171 = property class="VI"(reference=w360, error in=w359) -> (reference out=w357:refnum<vi>, error out=w358:errorcluster, "FP.State"=w356:T3)
            n172 = Not Equal?(x=w356, y=w354) -> (x != y?=w355:bool)
            n173 = case shown="True" w355 {
              tunnel: [w365 w366] -> w361
              tunnel: w358 -> [w364 w366]
              tunnel: w357 -> [w363 _]
              tunnel: w354 -> [w362 _]
              frame True {
                n174 = invoke class="VI" method="FP.Open"(reference=w363, error in=w364, "State"=w362) -> (error out=w365:errorcluster)  [unwired: 2 in, 4 out]
              }
              frame False {
              }
            }
          }
          frame "Minimize", "Minimized" {
            w367 = T3."Minimized" ("State")
            n175 = property class="VI"(reference=w373, error in=w372) -> (reference out=w370:refnum<vi>, error out=w371:errorcluster, "FP.State"=w369:T3)
            n176 = Not Equal?(x=w369, y=w367) -> (x != y?=w368:bool)
            n177 = case shown="True" w368 {
              tunnel: [w378 w379] -> w374
              tunnel: w371 -> [w377 w379]
              tunnel: w370 -> [w376 _]
              tunnel: w367 -> [w375 _]
              frame True {
                n178 = invoke class="VI" method="FP.Open"(reference=w376, error in=w377, "State"=w375) -> (error out=w378:errorcluster)  [unwired: 2 in, 4 out]
              }
              frame False {
              }
            }
          }
          frame "Maximize", "Maximized" {
            w380 = T3."Maximized" ("State")
            n179 = property class="VI"(reference=w386, error in=w385) -> (reference out=w383:refnum<vi>, error out=w384:errorcluster, "FP.State"=w382:T3)
            n180 = Not Equal?(x=w382, y=w380) -> (x != y?=w381:bool)
            n181 = case shown="True" w381 {
              tunnel: [w391 w392] -> w387
              tunnel: w384 -> [w390 w392]
              tunnel: w383 -> [w389 _]
              tunnel: w380 -> [w388 _]
              frame True {
                n182 = invoke class="VI" method="FP.Open"(reference=w389, error in=w390, "State"=w388) -> (error out=w391:errorcluster)  [unwired: 2 in, 4 out]
              }
              frame False {
              }
            }
          }
        }
        n183 = call <vilib>:"Add State(s) to Queue__jki_lib_state_machine.vi"("State(s) in (\"\")"=w327) -> ("States Out"=w326:string)  [unwired: 14 in]
      }
      frame "---------- Macro ----------" {
        # "Do not put any code in this frame.\n(It is a separator no-op. You can make a copy of this frame to create a new Macro frame)"
        n184 = call <vilib>:"Add State(s) to Queue__jki_lib_state_machine.vi"("State(s) in (\"\")"=w396) -> ("States Out"=w395:string)  [unwired: 14 in]
      }
      frame "Macro: Initialize" {
        w397 = "Data: Initialize\nInitialize Core Data\nUI: Initialize\nUI: Front Panel State >> Maximize\nCommunication: Open Serial\nCommunication: 读运行标志"  # Data: Initialize Initialize Core Data UI: Initialize UI: Front Panel State >> Maximize Communication: Open Serial Communication: 读运行标志
        # "Initialization Macro\n(This is called once, when the VI starts)"
        n185 = call <vilib>:"Add State(s) to Queue__jki_lib_state_machine.vi"("State(s) in Front (\"\")"=w397, "State(s) in (\"\")"=w401) -> ("States Out"=w400:string)  [unwired: 13 in]
      }
      frame "Macro: Exit" {
        # "Exit Macro\n(This is called once, when the VI exits)"
        n186 = Unbundle By Name(w408) -> ("Core.Close Panel on Exit?"=w407:bool)
        n187 = disable-structure shown="禁用" {
          frame Disabled {
            n188 = call "mes~设备状态采集.vi"("设备状态"="SHUTDOWN") -> ()  [unwired: 8 in, 3 out]
          }
          frame Enabled {
          }
        }
        n189 = Select(t="UI: Front Panel State >> Close", s=w407, f="") -> (s? t:f=w404:string)
        n190 = call <vilib>:"Add State(s) to Queue__jki_lib_state_machine.vi"("State(s) in (\"\")"=w404, "State(s) at Back (\"\")"="Data: Cleanup\nExit") -> ("States Out"=w402:string)  [unwired: 13 in]
        n191 = call <vilib>:"Add State(s) to Queue__jki_lib_state_machine.vi"("State(s) in Front (\"\")"=w402, "State(s) in (\"\")"=w411) -> ("States Out"=w410:string)  [unwired: 13 in]
      }
      frame "---------- Communication ----------" {
        # "Template Separator\n(You can make a copy of, or modify, this frame)"
        n192 = call <vilib>:"Add State(s) to Queue__jki_lib_state_machine.vi"("State(s) in (\"\")"=w416) -> ("States Out"=w415:string)  [unwired: 14 in]
      }
      frame "Communication: Open Serial" {
        # "Your code here.\n(You can make a copy of, or modify, this frame)"
        n193 = call "读取配置文件.vi"("error in"=w429, "配置"="串口号") -> ("error out"=w428:errorcluster, "路径"=w427:string)  [unwired: 8 in]
        n194 = call "开机连接.vi"("error in"=w428, "波特率"=u32 19200, "串口号"=w427) -> ("error out"=w421:errorcluster, "连接成功"=w423:bool, "serial master instance"=w425:refnum<class "Modbus Master.lvclass">)  [unwired: 6 in]
        n195 = disable-structure shown="Enabled" {
          disable-tunnel: [w440 _] -> w422
          disable-tunnel: w421 -> [w439 _]
          disable-tunnel: "温湿度" ("配置") -> [w438 _]
          disable-tunnel: [w434 _] -> w418
          disable-tunnel: [w433 TRUE ("连接成功")] -> w417
          frame Disabled {
            n196 = call "读取配置文件.vi"("error in"=w439, "配置"=w438) -> ("error out"=w437:errorcluster, "路径"=w436:string)  [unwired: 8 in]
            n197 = disable-structure shown="Enabled" {
              disable-tunnel: [u32 9600 ("波特率") u32 4800 ("波特率")] -> w435
              frame Disabled {
                # "箱体"
              }
              frame Enabled {
                # "液冷"
              }
            }
            n198 = call "开机连接.vi"("error in"=w437, "波特率"=w435, "串口号"=w436) -> ("error out"=w440:errorcluster, "连接成功"=w433:bool, "serial master instance"=w434:refnum<class "Modbus Master.lvclass">)  [unwired: 6 in]
          }
          frame Enabled {
          }
        }
        n199 = Bundle By Name(cluster=w426, "serial master instance"=w425, "连接成功"=w423, "温度instance"=w418) -> (w424:T7)
        n200 = case shown="True" w417 {
          frame False {
            n201 = One Button Dialog(message="温度串口连接失败。" ("消息")) -> ()  [unwired: 1 in, 1 out]
          }
          frame True {
          }
        }
        n202 = call <vilib>:"Add State(s) to Queue__jki_lib_state_machine.vi"("State(s) in (\"\")"=w432) -> ("States Out"=w431:string)  [unwired: 14 in]
      }
      frame "Communication: 设备启动" {
        w445 = TRUE
        # "Your code here.\n(You can make a copy of, or modify, this frame)"
        n203 = Unbundle By Name(w451) -> ("serial master instance"=w452:refnum<class "Modbus Master.lvclass">, "连接成功"=w453:bool)  [unwired: 2 out]
        n204 = And(x=w445, y=w445) -> (x .and. y?=w447:bool)
        n205 = case shown="False" w447 {
          tunnel: w455 -> [w460 w472]
          tunnel: [w460 w471] -> w454
          tunnel: w453 -> [w461 w470]
          tunnel: w452 -> [_ w469]
          tunnel: [w461 w468] -> w450
          tunnel: FALSE ("正在运行") -> [w462 w467]
          tunnel: [w462 w466] -> w446
          tunnel: w445 -> [w459 _]
          tunnel: w445 -> [w458 _]
          frame False {
            n206 = case shown="True" w459 {
              tunnel: w458 -> [_ w464]
              frame False {
                n207 = One Button Dialog(message="用户未登录。" ("消息")) -> ()  [unwired: 1 in, 1 out]
              }
              frame True {
                n208 = case shown="False" w464 {
                  frame False {
                    n209 = One Button Dialog(message="产品未进站。" ("消息")) -> ()  [unwired: 1 in, 1 out]
                  }
                  frame True {
                  }
                }
              }
            }
          }
          frame True {
            n210 = case shown="False" w467 {
              selector: w467 -> [_ w492]
              tunnel: w472 -> [w478 w493]
              tunnel: [w477 w493] -> w471
              tunnel: w470 -> [w476 w494]
              tunnel: w469 -> [w475 _]
              tunnel: [w474 w494] -> w468
              tunnel: [w473 w492] -> w466
              frame False {
                n211 = case shown="True" w476 {
                  tunnel: w478 -> [w479 w484]
                  tunnel: [w479 w483] -> w477
                  tunnel: w475 -> [_ w482]
                  tunnel: [_ w481] -> w474
                  tunnel: [_ TRUE] -> w473
                  frame False {
                  }
                  frame True {
                    n212 = stacked-sequence {
                      tunnel: w484 -> [_ w490 _]
                      tunnel: [_ w489 _] -> w483
                      tunnel: w482 -> [_ w488 _]
                      tunnel: [_ w487 _] -> w481
                      frame #0 {
                        n213 = local write "阻断通讯"(TRUE ("阻断通讯")) -> ()
                      }
                      frame #1 {
                        w486 = cluster{"地址":u16, "布尔":bool, "名称":string}[] [{"地址"=50, "布尔"=TRUE, "名称"="启动"}, {"地址"=51, "布尔"=FALSE, "名称"="停止"}]  # A写入线圈信息组
                        n214 = call "写入单个线圈.vi"("error in"=w490, "写入线圈信息组"=w486, "MB_实体"=w488) -> ("输出簇"=w489:errorcluster, "连接成功"=w487:bool)  [unwired: 7 in]
                      }
                      frame #2 {
                        n215 = local write "阻断通讯"(FALSE ("阻断通讯")) -> ()
                      }
                    }
                  }
                }
              }
              frame True {
              }
            }
          }
        }
        n216 = Bundle By Name(cluster=w451, "正在运行"=w446, "连接成功"=w450) -> (w449:T7)
        n217 = call <vilib>:"Add State(s) to Queue__jki_lib_state_machine.vi"("State(s) in (\"\")"=w457) -> ("States Out"=w456:string)  [unwired: 14 in]
      }
      frame "Communication: 设备停止" {
        # "Your code here.\n(You can make a copy of, or modify, this frame)"
        n218 = Unbundle By Name(w500) -> ("serial master instance"=w501:refnum<class "Modbus Master.lvclass">, "连接成功"=w502:bool)  [unwired: 1 out]
        n219 = case shown="True" TRUE ("正在运行") {
          tunnel: w504 -> [w509 w517]
          tunnel: [w509 w516] -> w503
          tunnel: w502 -> [w507 w515]
          tunnel: w501 -> [_ w514]
          tunnel: [w507 w513] -> w499
          tunnel: TRUE ("正在运行") -> [w508 w512]
          tunnel: [w508 w511] -> w497
          frame False {
            n220 = One Button Dialog(message="用户未登录" ("消息")) -> ()  [unwired: 1 in, 1 out]
          }
          frame True {
            n221 = case shown="True" w512 {
              selector: w512 -> [w518 _]
              tunnel: w517 -> [w519 w526]
              tunnel: [w519 w525] -> w516
              tunnel: w515 -> [w520 w524]
              tunnel: w514 -> [_ w523]
              tunnel: [w520 w522] -> w513
              tunnel: [w518 w521] -> w511
              frame False {
              }
              frame True {
                n222 = case shown="True" w524 {
                  tunnel: w526 -> [w528 w533]
                  tunnel: [w528 w532] -> w525
                  tunnel: w523 -> [_ w531]
                  tunnel: [_ w530] -> w522
                  tunnel: [FALSE FALSE] -> w521
                  frame False {
                  }
                  frame True {
                    n223 = stacked-sequence {
                      tunnel: w533 -> [_ w539 _]
                      tunnel: [_ w538 _] -> w532
                      tunnel: w531 -> [_ w537 _]
                      tunnel: [_ w536 _] -> w530
                      frame #0 {
                        n224 = local write "阻断通讯"(TRUE ("阻断通讯")) -> ()
                      }
                      frame #1 {
                        w535 = cluster{"地址":u16, "布尔":bool, "名称":string}[] [{"地址"=50, "布尔"=FALSE, "名称"="启动"}, {"地址"=51, "布尔"=TRUE, "名称"="停止"}]  # A写入线圈信息组
                        n225 = call "写入单个线圈.vi"("error in"=w539, "写入线圈信息组"=w535, "MB_实体"=w537) -> ("输出簇"=w538:errorcluster, "连接成功"=w536:bool)  [unwired: 7 in]
                      }
                      frame #2 {
                        n226 = local write "阻断通讯"(FALSE ("阻断通讯")) -> ()
                      }
                    }
                  }
                }
              }
            }
          }
        }
        n227 = Bundle By Name(cluster=w500, "正在运行"=w497, "连接成功"=w499) -> (w498:T7)
        n228 = call <vilib>:"Add State(s) to Queue__jki_lib_state_machine.vi"("State(s) in (\"\")"=w506) -> ("States Out"=w505:string)  [unwired: 14 in]
      }
      frame "Communication: 读运行标志" {
        n229 = Unbundle By Name(w542) -> ("serial master instance"=w541:refnum<class "Modbus Master.lvclass">)
        n230 = stacked-sequence {
          tunnel: w547 -> [_ w556 _]
          tunnel: [_ w555 _] -> w546
          tunnel: [_ w554 _] -> w545
          tunnel: [_ w553 _] -> w544
          tunnel: w541 -> [_ w551 _]
          frame #0 {
            n231 = local write "阻断通讯"(TRUE ("阻断通讯")) -> ()
          }
          frame #1 {
            w552 = T9 [{"地址"=507, "数量"=1, "名称"="1测试结束标志", "线圈组"=[]}]  # A读多组线圈信息组
            n232 = call "读线圈组.vi"("error in"=w556, "读多组线圈__输入"=w552, "MB_实体"=w551) -> ("输出簇"=w555:errorcluster, "正在运行"=w553:bool, "连接成功"=w554:bool)  [unwired: 6 in]
          }
          frame #2 {
            n233 = local write "阻断通讯"(FALSE ("阻断通讯")) -> ()
          }
        }
        n234 = Bundle By Name(cluster=w542, "连接成功"=w545, "正在运行"=w544) -> (w543:T7)
        n235 = call <vilib>:"Add State(s) to Queue__jki_lib_state_machine.vi"("State(s) in (\"\")"=w549) -> ("States Out"=w548:string)  [unwired: 14 in]
      }
      frame "---------- 设备状态采集 ----------" {
        # "Do not put any code in this frame.\n(it is a separator no-op)"
        n236 = call <vilib>:"Add State(s) to Queue__jki_lib_state_machine.vi"("State(s) in (\"\")"=w561) -> ("States Out"=w560:string)  [unwired: 14 in]
      }
      frame "通讯参数设置" {
        n237 = stacked-sequence {
          tunnel: w563 -> [_ w571 _]
          tunnel: [_ w568 _] -> w562
          frame #0 {
            n238 = local write "阻断通讯"(TRUE ("阻断通讯")) -> ()
          }
          frame #1 {
            n239 = call "通讯参数设置.vi"() -> ("A设备簇"=w572:T8)  [unwired: 5 in]
            n240 = Unbundle By Name(w572) -> ("MB_实体"=w570:refnum<class "Modbus Master.lvclass">, "连接成功"=w569:bool)
            n241 = Bundle By Name(cluster=w571, "serial master instance"=w570, "连接成功"=w569) -> (w568:T7)
          }
          frame #2 {
            n242 = local write "阻断通讯"(FALSE ("阻断通讯")) -> ()
          }
        }
        n243 = call <vilib>:"Add State(s) to Queue__jki_lib_state_machine.vi"("State(s) in (\"\")"=w566) -> ("States Out"=w565:string)  [unwired: 14 in]
      }
    }
  }
